vi "setIDs.vi"(8 "error in (no error)":errorcluster, 10 "IDs":u32[](array[numeric]), 11 "LLNode in":refnum<class "LLNode.lvclass">) -> (0 "error out":errorcluster, 3 "LLNode out":refnum<class "LLNode.lvclass">)   [LabVIEW 2009, in "LLNode.lvclass"]
uses:
  LLNode.lvclass
  Node/Node.lvclass
  LLNode.lvclass/LLNode.ctl
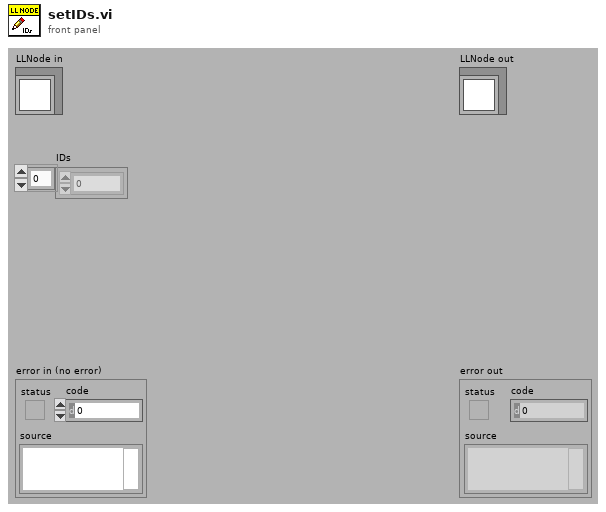
[diagram p1: front panel]
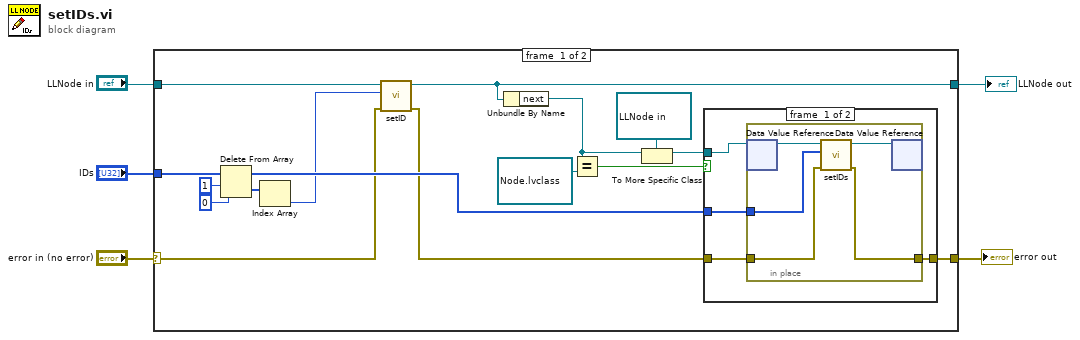
[diagram p0: block diagram]
diagram:
  n1 = case shown="No Error" "error in (no error)" {
    selector: "error in (no error)" -> [w7 w32]
    tunnel: [w11 w32] -> w2
    tunnel: [w9 w33] -> w1
    tunnel: "LLNode in" -> [w10 w33]
    tunnel: "IDs" -> [w21 _]
    frame #0 {
      n2 = Delete From Array(array=w21, length=1, index=0) -> (deleted portion=w18:u32[], array with subset deleted=w12:u32[])
      n3 = Index Array(array=w18) -> (element=w8:u32)  [unwired: 1 in]
      n4 = call "setID.vi"("error in (no error)"=w7, "ID"=w8, "Node in"=w10) -> ("error out"=w6:errorcluster, "Node out"=w9:refnum<class "LLNode.lvclass">)  [unwired: 7 in]
      n5 = Unbundle By Name(w9) -> ("next"=w13:refnum<data-value>)
      n6 = Equal?(x=w13, y=refnum<data-value> refnum) -> (x = y?=w16:bool)
      n7 = To More Specific Class(target class=refnum<data-value> refnum ("data value reference"), reference=w13) -> (specific class reference=w15:refnum<data-value>)  [unwired: 1 in, 1 out]
      n8 = case shown="False" w16 {
        tunnel: w12 -> [w23 _]
        tunnel: w15 -> [w25 _]
        tunnel: w6 -> [w24 w31]
        tunnel: [w22 w31] -> w11
        frame #0 {
          n9 = in-place {
            in-place-border: w24 -> [w30]
            in-place-border: w23 -> [w29]
            in-place-border: [w28] -> w22
            n10 = in-place-dvr #1(w25) -> (w26:refnum<class "LLNode.lvclass">)  [unwired: 1 out]
            n11 = call "setIDs.vi"("error in (no error)"=w30, "IDs"=w29, "LLNode in"=w26) -> ("error out"=w28:errorcluster, "LLNode out"=w27:refnum<class "LLNode.lvclass">)  [unwired: 7 in]
            n12 = in-place-dvr #1(w27) -> ()  [unwired: 2 out]
          }
        }
        frame #1 {
        }
      }
    }
    frame #1 {
    }
  }
  "error out" <- w2
  "LLNode out" <- w1
